vi "Set Color.vi"(8 "Color":u32(colorbox), 11 "Point In":refnum<class "Point.lvclass">) -> (3 "Point Out":refnum<class "Point.lvclass">)   [LabVIEW 2019, in "Point.lvclass"]
doc: "Set the point's color."
uses:
  Point.lvclass
  e:/builds/penguin/labview/branches/2019/dev/dist/examples/Object-Oriented Programming/Graphics/Graphic/Graphic.lvclass
  Point.lvclass/Point.ctl
  Graphic/Graphic.lvclass
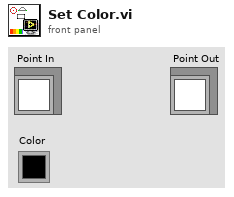
[diagram p1: front panel]
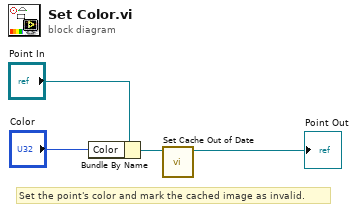
[diagram p0: block diagram]
diagram:
  # "Set the point's color and mark the cached image as invalid."
  n1 = Bundle By Name(cluster="Point In", "Color"="Color") -> (w2:refnum<class "Point.lvclass">)
  n2 = call "Set Cache Out of Date.vi"("Graphic.lvclass"=w2) -> ("Graphic.lvclass out"=→"Point Out":refnum<class "Point.lvclass">)  [unwired: 10 in]
